vi "Configure Basic PID Parameters.vi"(0 "VISA resource name":refnum<visa-resource-name>, 1 "Unit Address (1)":u8=1 min=1 max=254, 7 "Proportional Band (1)":sgl=1.0 min=0.1 max=3000, 9 "Integral Time (1)":i32=1 min=0 max=9999, 11 "error in (no error)":errorcluster, 12 "Derivative Time (0)":i32 min=0 max=9999) -> (4 "VISA resource name out":refnum<visa-resource-name>, 15 "error out":errorcluster)   [LabVIEW 2010, in "Eurotherm 32xx Series.lvlib"]
doc: "This VI sets basic PID parameters."
uses:
  <instrlib>/Eurotherm 32xx Series/Eurotherm 32xx Series.lvlib
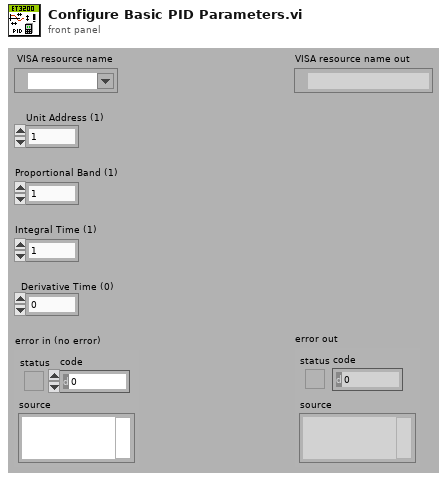
[diagram p1: front panel]
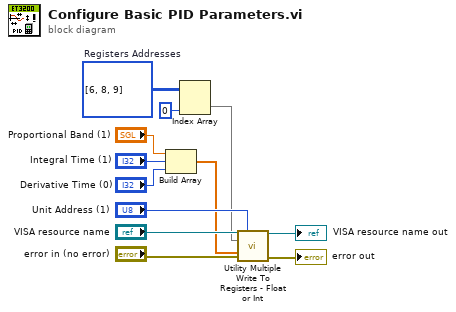
[diagram p0: block diagram]
diagram:
  w12 = u16[][] [[6], [8], [9]]  # Registers Addresses
  n1 = Build Array("Proportional Band (1)", "Integral Time (1)", "Derivative Time (0)") -> (w2:sgl[])
  n2 = Index Array(array=w12, index (col)=0 ("Number of PID (1)")) -> (element=w3:u16[])  [unwired: 1 in]
  n3 = call <instrlib>:"Utility Multiple Write To Registers - Float or Int.vi"("VISA resource name"="VISA resource name", "Unit Address (1)"="Unit Address (1)", "Registers Addresses (0)"=w3, "Data (0)"=w2, "error in (no error)"="error in (no error)") -> ("VISA resource name out"=→"VISA resource name out":refnum<visa-resource-name>, "error out"=→"error out":errorcluster)  [unwired: 9 in]
